vi "Write Element of Frequency.vi"(8 "error in (no error)":errorcluster, 9 "frequency (1000.0 Hz)":dbl[unit]=1000.0 format="%^.2e", 10 "index":i32, 11 "CS++FgenChannelData in":refnum<class "CS++FgenChannelData.lvclass">) -> (0 "error out":errorcluster, 3 "CS++FgenChannelData out":refnum<class "CS++FgenChannelData.lvclass">)   [LabVIEW 2013, in "CS++FgenGui.lvlib" / "CS++FgenChannelData.lvclass"]
uses:
  CS++FgenChannelData.lvclass
  CS++FgenChannelData.lvclass/CS++FgenChannelData.ctl
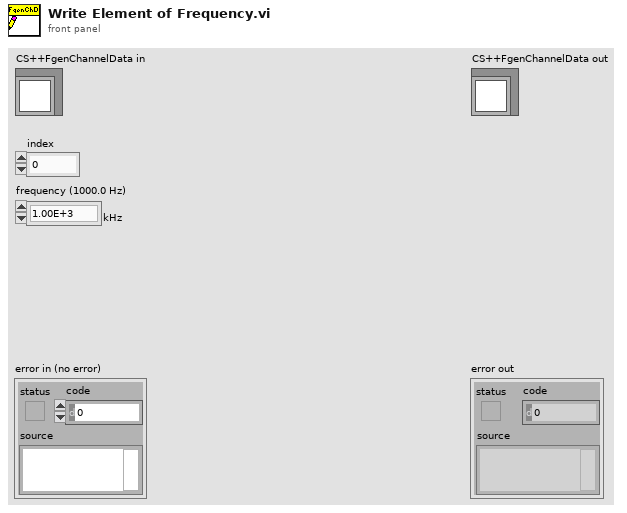
[diagram p1: front panel]
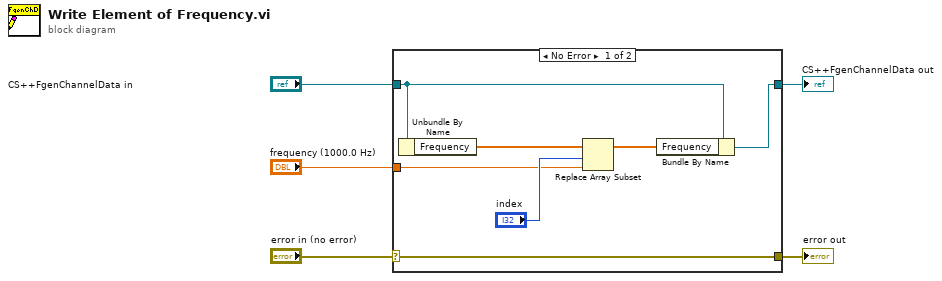
[diagram p0: block diagram]
diagram:
  n1 = case shown="No Error" "error in (no error)" {
    selector: "error in (no error)" -> [w12 w13]
    tunnel: [w12 w13] -> w4
    tunnel: [w11 w14] -> w2
    tunnel: "CS++FgenChannelData in" -> [w10 w14]
    tunnel: "frequency (1000.0 Hz)" -> [w6 _]
    frame No Error {
      n2 = Unbundle By Name(w10) -> ("Frequency"=w9:dbl[unit][])
      n3 = Replace Array Subset(array=w9, new element=w6, index="index") -> (w8:dbl[unit][])
      n4 = Bundle By Name(cluster=w10, "Frequency"=w8) -> (w11:refnum<class "CS++FgenChannelData.lvclass">)
    }
    frame Error {
    }
  }
  "error out" <- w4
  "CS++FgenChannelData out" <- w2
